vi "Keithley 197A read.vi"(8 "error in (no error)":errorcluster, 11 "VISA resource name":refnum<visa-resource-name>) -> (0 "error out":errorcluster, 3 "Numeric Output":dbl format="%.5f")   [LabVIEW 2015]
panel:
  out "read buffer":string
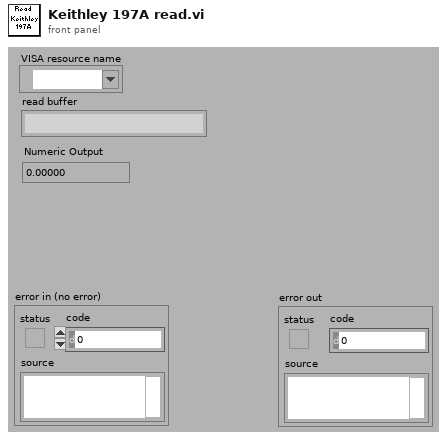
[diagram p1: front panel]
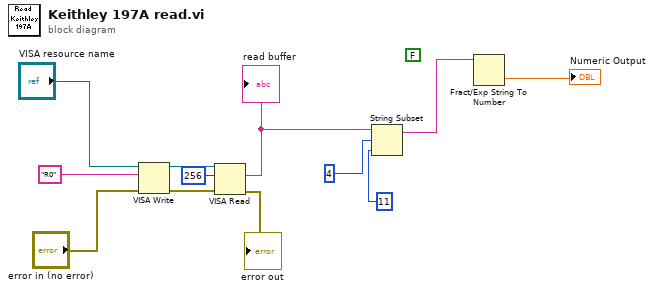
[diagram p0: block diagram]
diagram:
  (unwired) FALSE ("use system decimal point (T)")
  n1 = VISA Write(VISA resource name="VISA resource name", write buffer="R0", error in (no error)="error in (no error)") -> (VISA resource name out=w8:refnum<visa-resource-name>, error out=w11:errorcluster)  [unwired: 1 out]
  n2 = VISA Read(VISA resource name=w8, byte count=u32 256, error in (no error)=w11) -> (read buffer=w2:string, error out=→"error out":errorcluster)  [unwired: 2 out]
  "read buffer" <- w2
  n3 = String Subset(string=w2, offset (0)=4, length (rest)=11) -> (substring=w6:string)
  n4 = Fract/Exp String To Number(string=w6) -> (number=→"Numeric Output":dbl)  [unwired: 4 out]
